vi "PE Get System Count.vi"(8 "error in (no error)":errorcluster, 11 "peHandle":u32) -> (0 "error out":errorcluster, 3 "function return":i32)   [LabVIEW 2017, in "PE_Filter_SDK.lvlib"]
doc: "PEFILTERSDK_API int PE_GetSystemCount(CPE_HANDLE peHandle);"
uses:
  PE_Filter_SDK.lvlib
  PE_Filter_SDK.dll
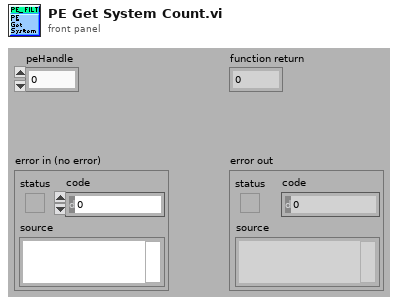
[diagram p1: front panel]
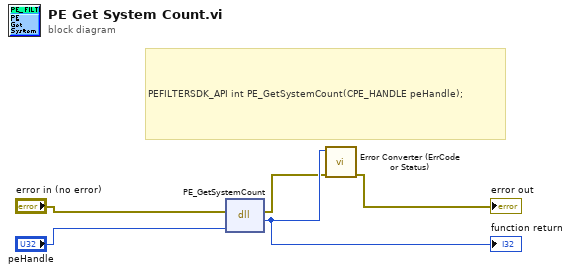
[diagram p0: block diagram]
diagram:
  # "PEFILTERSDK_API int PE_GetSystemCount(CPE_HANDLE peHandle);"
  n1 = dll-call lib="D:/working_directory/SDK LLTF/trunk_commit/examples/PE_Filter_SDK/PE_Filter_SDK.*" fn="PE_GetSystemCount"(error in="error in (no error)", "peHandle"="peHandle") -> (error out=w2:errorcluster, w5:i32)  [unwired: 3 in, 1 out]
  "function return" <- w5
  n2 = call "Error Converter (ErrCode or Status).vi"("error in (no error)"=w2, "error code"=w5) -> ("error out"=→"error out":errorcluster)  [unwired: 9 in]
